vi "Esercitazione 3 - Esercizio per casa, valore intermedio.vi"() -> ()   [LabVIEW 2018]
panel:
  out "Numeric Indicator":dbl
  in  "C":dbl
  in  "B":dbl
  in  "A":dbl
  # "dati tre valori numerici, restituire  il valore intermedio"
  # "suggerimento = case structure"
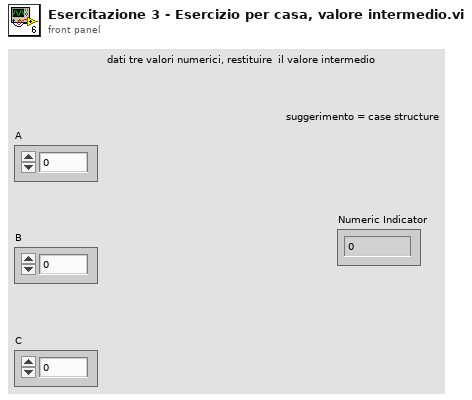
[diagram p1: front panel]
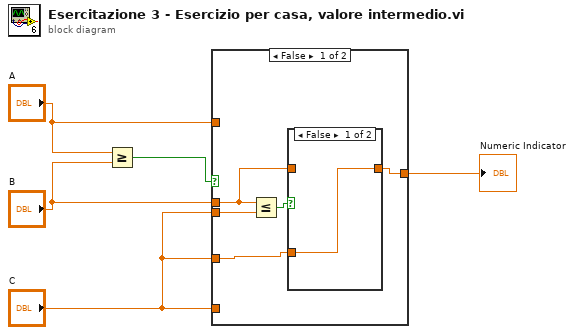
[diagram p0: block diagram]
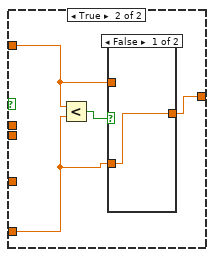
[diagram p3: hidden frame]
diagram:
  n1 = Greater Or Equal?(x="A", y="B") -> (x >= y?=w5:bool)
  n2 = case shown="False" w5 {
    tunnel: "A" -> [_ w15]
    tunnel: "C" -> [_ w13]
    tunnel: [w8 w14] -> w3
    tunnel: "B" -> [w9 _]
    tunnel: "C" -> [w7 _]
    tunnel: "C" -> [w6 _]
    frame False {
      n3 = Less Or Equal?(x=w9, y=w7) -> (x <= y?=w10:bool)
      n4 = case shown="False" w10 {
        tunnel: w9 -> [_ w12]
        tunnel: [w11 w12] -> w8
        tunnel: w6 -> [w11 _]
        frame False {
        }
        frame True {
        }
      }
    }
    frame True {
      n5 = Less?(x=w15, y=w13) -> (x < y?=w16:bool)
      n6 = case shown="False" w16 {
        tunnel: [w17 w18] -> w14
        tunnel: w15 -> [_ w18]
        tunnel: w13 -> [w17 _]
        frame False {
        }
        frame True {
        }
      }
    }
  }
  "Numeric Indicator" <- w3
